vi "MarkerSkill.vi"(5 "SecondMostDangerous":bool, 7 "firstCall":bool, 8 "error in (no error)":errorcluster, 9 "Robot":refnum<class "Robot.lvclass">, 10 "Game":refnum<class "Game.lvclass">, 11 "MarkerSkill in":refnum<class "MarkerSkill.lvclass">) -> (0 "error out":errorcluster, 2 "Robot out":refnum<class "Robot.lvclass">, 3 "MarkerSkill out":refnum<class "MarkerSkill.lvclass">)   [LabVIEW 2020, in "MarkerSkill.lvclass"]
uses:
  MarkerSkill.lvclass
  Robot_class/Robot.lvclass
  Game_class/Game.lvclass
  Utilities_class/Utilities.lvclass
  Referee_class/command_interpreted.ctl
  Team_class/OffensivePlay.ctl
  Game_class/Game.lvclass/Game.ctl
  Team_class/Team.lvclass/Team.ctl
  Object_class/Object.lvclass/Object.ctl
  Parameters_class/Parameters.lvclass/Parameters.ctl
  Referee_class/Referee.lvclass/Referee.ctl
  Robot_class/Robot.lvclass/Robot.ctl
  Robot_class/roles.ctl
  Robot_class/Read role.vi
  Object_class/Read x.vi
  Object_class/Read y.vi
  Robot_class/Read id.vi
  <vilib>/Analysis/_algsub.llb/Real Vector Norm.vi
  Robot_class/Write dest_x.vi
  Robot_class/Write dest_y.vi
  Robot_class/Write dest_orientation.vi
  Robot_class/Write dest_vel.vi
  Robot_class/Read orientation.vi
  Game_class/Read BallRef.vi
  Game_class/Read Referee.vi
  Game_class/Read Parameters.lvclass.vi
  Parameters_class/Read DistanceStop.vi
  Referee_class/Read command_interpreted.vi
  Game_class/Read OffensiveTeam.vi
  Team_class/Read RobotRef.vi
  Game_class/Read EnemyRef.vi
  Game_class/Read Utilities.lvclass.vi
  Game_class/Read FieldRef.vi
  Parameters_class/Read Type of Marker.vi
  Team_class/Read OffensivePlay.vi
  Robot_class/Read dest_x.vi
  Robot_class/Read dest_y.vi
  Ball_class/Ball.lvclass
  Enemy_class/Enemy.lvclass
  Ally_class/Ally.lvclass
  Field_class/Field.lvclass
  Parameters_class/Parameters.lvclass
  Referee_class/Referee.lvclass
  <vilib>/Analysis/NI_AALPro.lvlib
panel:
  out "id do inimigo\nmais perigoso":u32
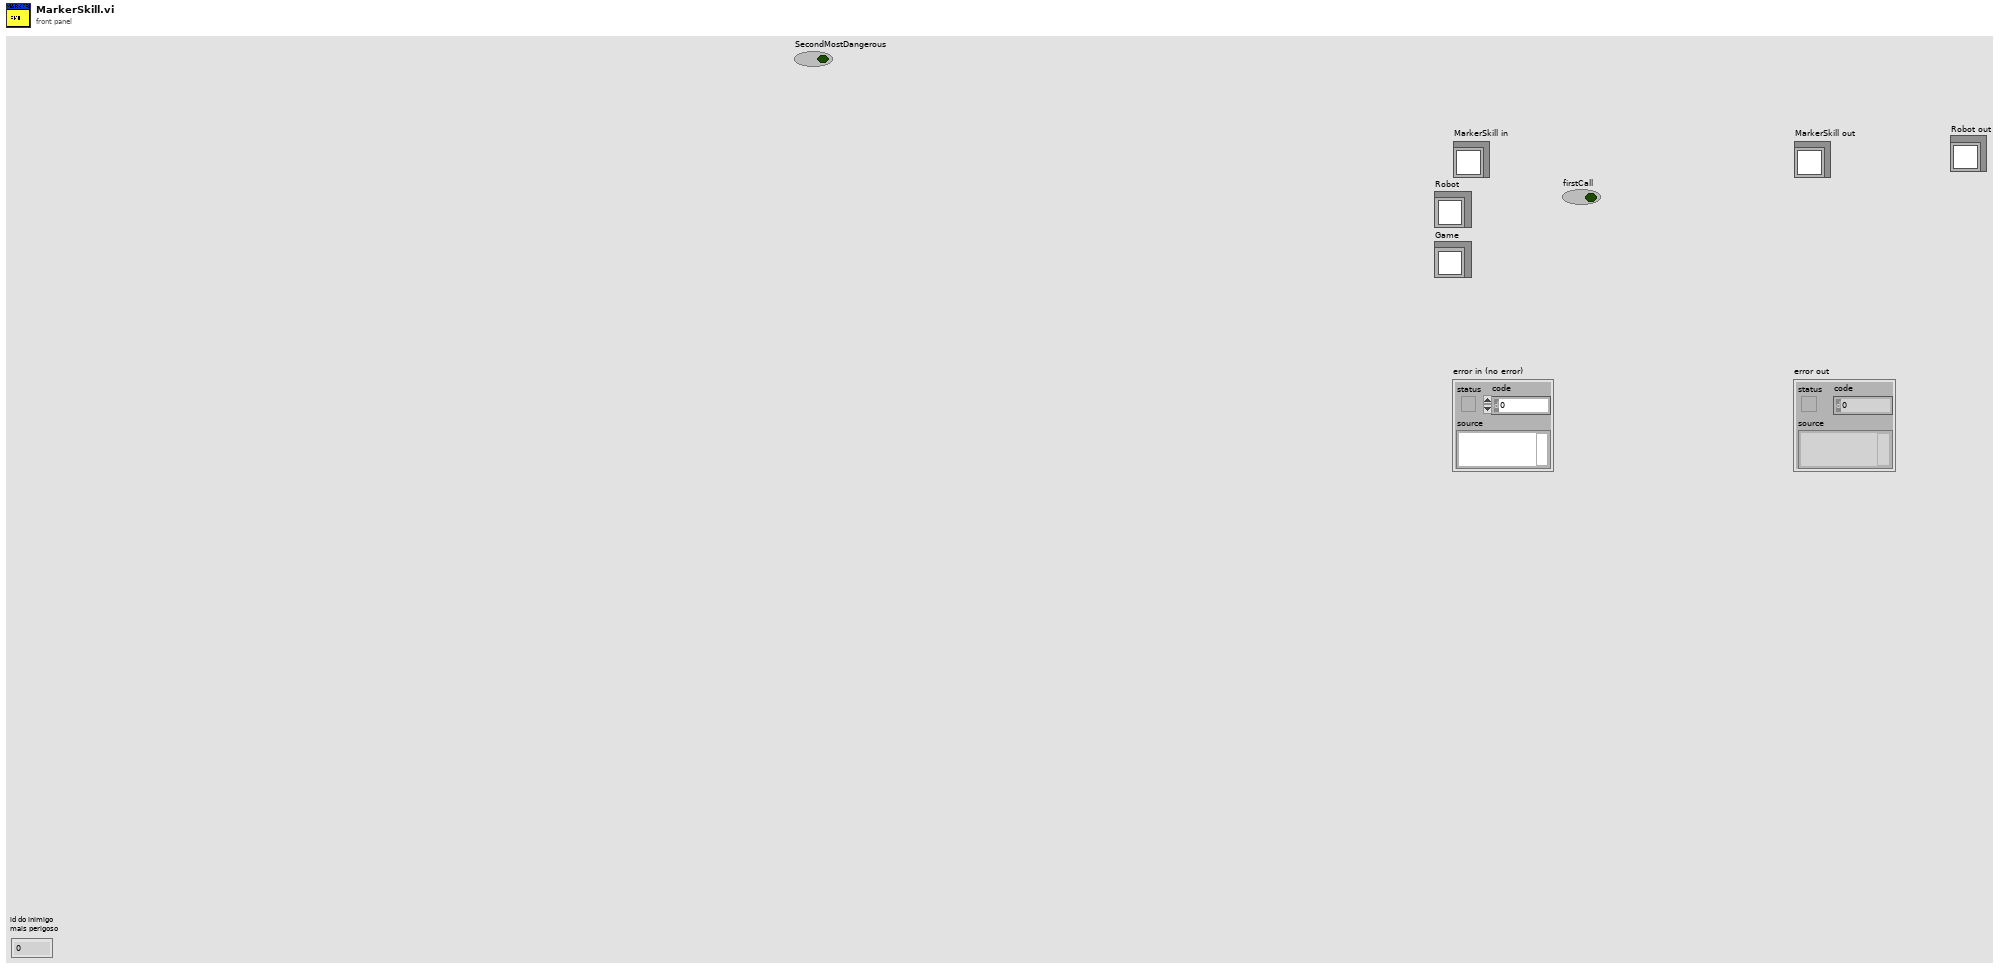
[diagram p1: front panel]
types:
  T1 = typedef "OffensivePlay.ctl" = enum16{"5RobotsPassGamePlay", "5PreparePassGame", "5RobotsKeeperGame", "KeeperPassToStriker", "5RobotsNormalGamePlay", "PrepareKeeperPass", "ACBPass", "ABCPass", "PrepareTriplePass", "TableWithStriker", "TableWith2ndStrikerPlay", "PrepareDoublePass", "PrepareRollToPass", "SimplePass", "PreparePass", "PassToStriker", "BallOutOfField", "PassTo2ndStriker", "StopOffensive", "Prepare Penalty Enemy", "EnemyPossessionAtEnemyField", "EnemyPossesionAtOurField", "TestPlay", "PreparePenaltyAlly", "KickPenaltyAlly", "PrepareKickoffAlly", "PrepareKickoffEnemy", "IndirectEnemy", "DirectEnemy", "PreparePassInGame1", "NormalGame", "DirectKick", "Pass", "Halt", "Timeout", "PassPlay", "PenaltyEnemy"}
  T2 = typedef "command_interpreted.ctl" = enum16{"Goal Ally", "Goal Enemy", "Ball Placement Enemy", "Ball Placement Ally", "Normal Half Time", "Extra Time  Break", "Extra Half Time", "None", "Post Game", "PKA Normal Start", "Prepare Kickoff Ally", "PKE Normal Start", "Prepare Kickoff Enemy", "Force Start", "Halt", "Timeout", "Prepare Penalty Ally", "Prepare Penalty Enemy", "PPA NormalStart", "PPE Normal Start", "Indirect Free Ally", "Direct Free Enemy", "Direct Free Ally", "Indirect Free Enemy", "Stop"}
  T3 = typedef "roles.ctl" = enum16{"SecondMarker", "5Robots5th", "PassBestReceiver", "5Robots4th", "5Robots3rd", "5Robots2nd", "5Robots1st", "PassBestRobot", "WaitPass", "ABCThirdKicker", "ABCFirstKicker", "ABCSecondKicker", "Tabler", "TableFinalizer", "PrepareRollToPassRoller", "PrepareRollToPassReceiver", "SimplePassRoll", "SimplePassRollReceiver", "PenaltyDefense", "PreparePassReceiver 2", "PreparePassReceiver 1", "PassObserver", "Timeout", "Goto", "ZigZag", "None", "BallOutOfField", "DefenderArea", "Duelist", "AttackerStop", "FollowAttacker", "KeeperRole", "KickPenalty", "AttackerAimGoal", "AttackerBlock", "Marker", "Halt", "Shoot", "PassKicker", "PassReceiver", "TestRole", "PenaltyAttacker"}
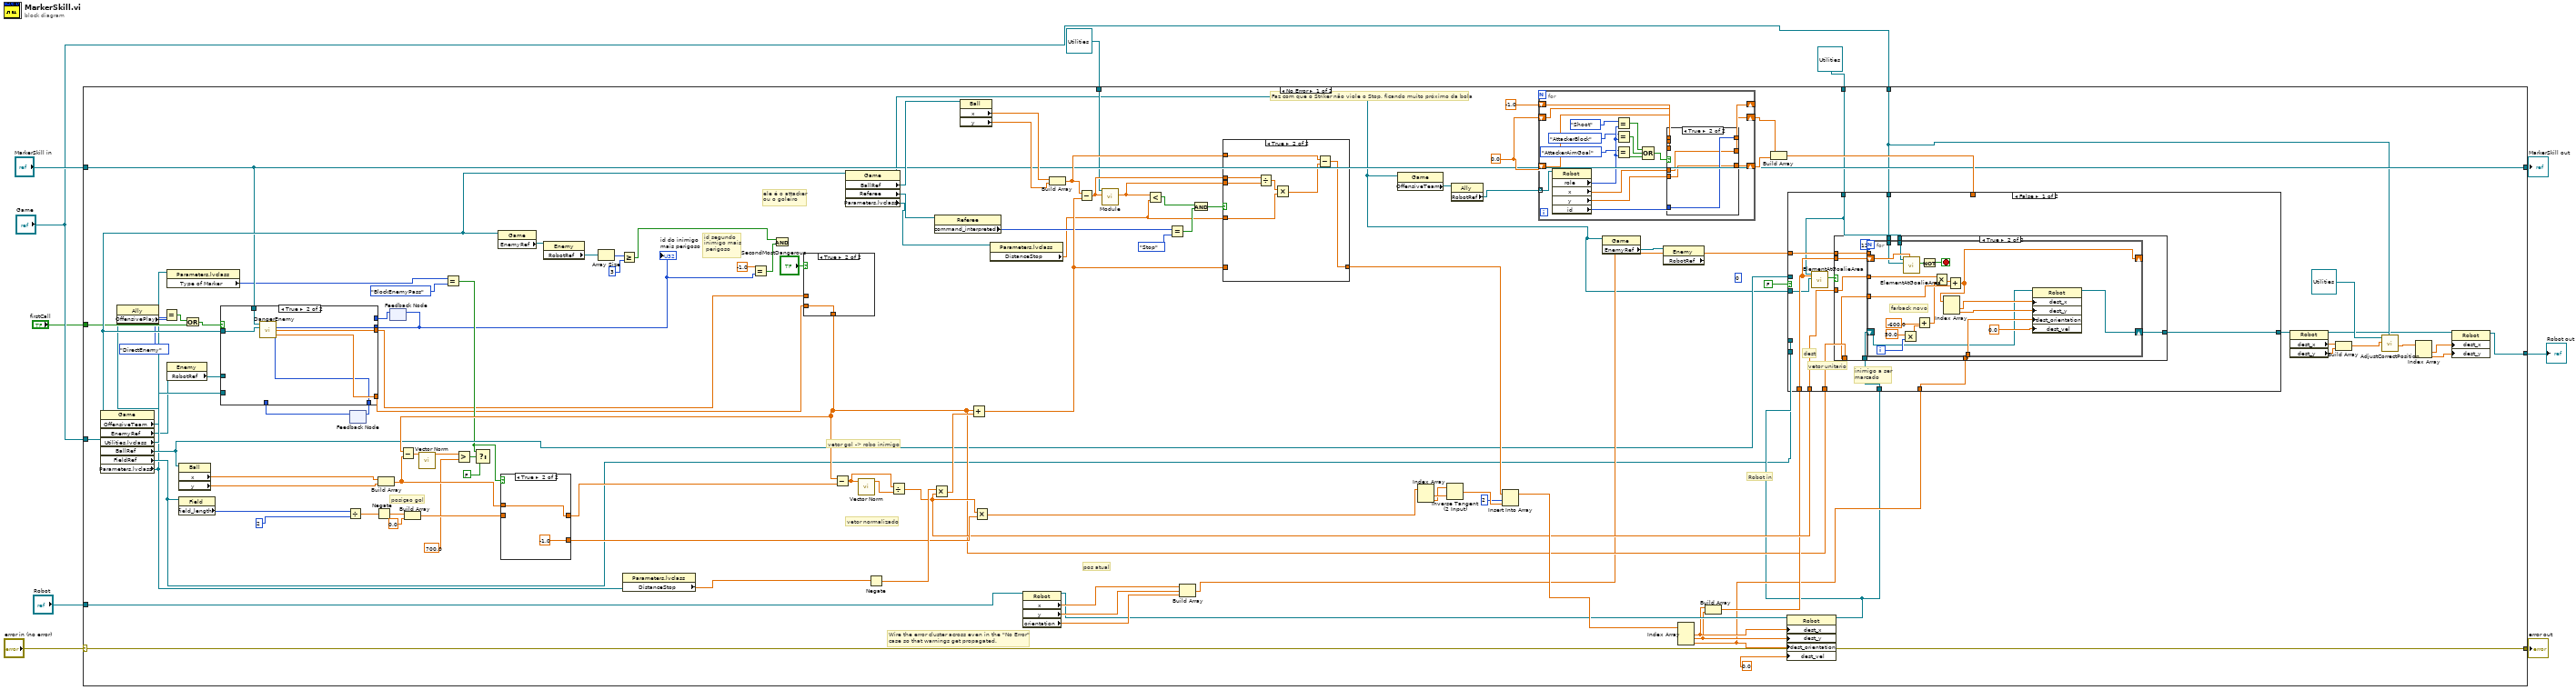
[diagram p0: block diagram]
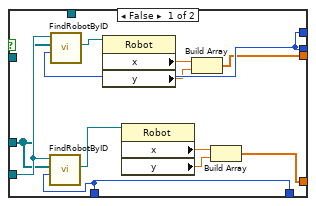
[diagram p2: hidden frame]
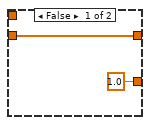
[diagram p7: hidden frame]
diagram:
  n1 = case shown="No Error" "error in (no error)" {
    selector: "error in (no error)" -> [w122 w222]
    tunnel: [w122 w222] -> w9
    tunnel: [w51 w221] -> w7
    tunnel: "MarkerSkill in" -> [w51 w221]
    tunnel: "Game" -> [w52 _]
    tunnel: "Robot" -> [w76 _]
    tunnel: refnum<class "Utilities.lvclass"> refnum ("Utilities in") -> [w48 _]
    tunnel: refnum<class "Utilities.lvclass"> refnum ("Utilities in") -> [w47 _]
    tunnel: "Game" -> [w26 _]
    tunnel: "firstCall" -> [w17 _]
    tunnel: [w22 _] -> w1
    frame No Error {
      (unwired) 0 ("y")
      w96 = 0.0
      # "id segundo \ninimigo mais\n perigoso"
      # "Robot in"
      # "ele é o attacker\nou o goleiro"
      # "Faz com que o Striker não viole o Stop, ficando muito próximo da bola"
      # "pos atual"
      # "vetor normalizado"
      # "vetor gol -> robo inimigo"
      # "posiçao gol"
      # "Wire the error cluster across even in the \"No Error\"\ncase so that warnings get propagated."
      n2 = property class="Game"(reference=w52) -> ("OffensiveTeam"=w16:refnum<class "Ally.lvclass">, "EnemyRef"=w32:refnum<class "Enemy.lvclass">, "Utilities.lvclass"=w33:refnum<class "Utilities.lvclass">, "BallRef"=w66:refnum<class "Ball.lvclass">, "FieldRef"=w54:refnum<class "Field.lvclass">, "Parameters.lvclass"=w12:refnum<class "Parameters.lvclass">)  [unwired: 1 in, 2 out]
      n3 = property class="Ally"(reference=w16) -> ("OffensivePlay"=w15:T1)  [unwired: 1 in, 2 out]
      n4 = Equal?(x=w15, y=OffensivePlay."DirectEnemy") -> (x = y?=w13:bool)
      n5 = property class="Enemy"(reference=w32) -> ("RobotRef"=w31:refnum<class "Robot.lvclass">[])  [unwired: 1 in, 2 out]
      n6 = property class="Parameters.lvclass"(reference=w12) -> ("Type of Marker"=w44:enum16{"BlockEnemyPass", "BlockOurGoal"})  [unwired: 1 in, 2 out]
      n7 = property class="Ball"(reference=w66) -> ("x"=w78:dbl, "y"=w77:dbl)  [unwired: 1 in, 2 out]
      n8 = property class="Field"(reference=w54) -> ("field_length"=w53:i32)  [unwired: 1 in, 2 out]
      n9 = Or(x=w13, y=w17) -> (x .or. y?=w18:bool)
      n10 = Divide(x=w53, y=u32 2) -> (x/y=w120:dbl)
      n11 = feedback #1() -> (w34:i32)  [unwired: 1 in]
      n12 = Negate(x=w120) -> (-x=w119:dbl)
      n13 = Build Array(w78, w77) -> (w89:dbl[])
      n14 = feedback #2() -> (w36:u32)  [unwired: 1 in]
      n15 = case shown="True" w18 {
        tunnel: [w133 w140] -> w37
        tunnel: [w127 w139] -> w38
        tunnel: [w123 w138] -> w39
        tunnel: w52 -> [_ w137]
        tunnel: w51 -> [_ w136]
        tunnel: w36 -> [w133 _]
        tunnel: [w131 w135] -> w35
        tunnel: w34 -> [w131 _]
        tunnel: w33 -> [w134 _]
        tunnel: w31 -> [w132 _]
        frame False {
          n16 = call "FindRobotByID.vi"("id"=w131, "RobotRef"=w132, "Utilities in"=w134) -> ("Robot"=w124:refnum<class "Robot.lvclass">)  [unwired: 5 in, 3 out]
          n17 = call "FindRobotByID.vi"("id"=w133, "RobotRef"=w132, "Utilities in"=w134) -> ("Robot"=w130:refnum<class "Robot.lvclass">)  [unwired: 5 in, 3 out]
          n18 = property class="Robot"(reference=w130) -> ("x"=w129:dbl, "y"=w128:dbl)  [unwired: 1 in, 2 out]
          n19 = property class="Robot"(reference=w124) -> ("x"=w126:dbl, "y"=w125:dbl)  [unwired: 1 in, 2 out]
          n20 = Build Array(w129, w128) -> (w127:dbl[])
          n21 = Build Array(w126, w125) -> (w123:dbl[])
        }
        frame True {
          n22 = call-dynamic "DangerEnemy.vi"("MarkerSkill in"=w136, "Game"=w137) -> ("id do inimigo\nmais perigoso"=w140:u32, "Pos do inimigo\nperigoso"=w139:dbl[], "id do segundo inimigo\nmais perigoso"=w135:i32, "Pos do segundo inimigo\nperigoso"=w138:dbl[])  [unwired: 6 in, 4 out]
        }
      }
      "id do inimigo\nmais perigoso" <- w37
      n23 = feedback-in #1(w35) -> ()
      n24 = feedback-in #2(w37) -> ()
      n25 = Build Array(w119, 0.0 ("element")) -> (w105:dbl[])
      n26 = Equal?(x=w44, y=enum16{"BlockEnemyPass", "BlockOurGoal"}."BlockEnemyPass" ("Type of Marker")) -> (x = y?=w45:bool)
      n27 = property class="Game"(reference=w52) -> ("EnemyRef"=w65:refnum<class "Enemy.lvclass">)  [unwired: 1 in, 2 out]
      n28 = case shown="True" w45 {
        tunnel: [w210 w211] -> w90
        tunnel: w105 -> [w210 _]
        tunnel: [1.0 -1.0] -> w101
        tunnel: w89 -> [_ w211]
        frame False {
        }
        frame True {
        }
      }
      n29 = property class="Enemy"(reference=w65) -> ("RobotRef"=w64:refnum<class "Robot.lvclass">[])  [unwired: 1 in, 2 out]
      n30 = Array Size(array=w64) -> (size(s)=w94:i32)
      n31 = Greater Or Equal?(x=w94, y=3) -> (x >= y?=w92:bool)
      n32 = property class="Parameters.lvclass"(reference=w12) -> ("DistanceStop"=w11:dbl)  [unwired: 1 in, 2 out]
      n33 = Equal?(x=-1.0, y=w37) -> (x = y?=w91:bool)
      n34 = And(x=w92, y=w91) -> ()  [unwired: 1 out]
      n35 = case shown="True" "SecondMostDangerous" {
        tunnel: w38 -> [w141 _]
        tunnel: w39 -> [_ w142]
        tunnel: [w141 w142] -> w80
        frame False {
        }
        frame True {
        }
      }
      n36 = Subtract(x=w80, y=w89) -> (x-y=w88:dbl[])
      n37 = call-poly <vilib>:"Vector Norm.vi"("Input Vector"=w88) -> ("norm"=w87:dbl)  [unwired: 9 in, 1 out]
      n38 = Greater?(x=w87, y=700.0) -> (0:w86:bool)
      n39 = Select(t=w45, s=w86, f=FALSE) -> ()  [unwired: 1 out]
      n40 = Subtract(x=w80, y=w90) -> (x-y=w116:dbl[])
      n41 = property class="Game"(reference=w52) -> (reference out=w40:refnum<class "Game.lvclass">, "BallRef"=w63:refnum<class "Ball.lvclass">, "Referee"=w60:refnum<class "Referee.lvclass">, "Parameters.lvclass"=w43:refnum<class "Parameters.lvclass">)  [unwired: 1 in, 1 out]
      n42 = call-poly <vilib>:"Vector Norm.vi"("Input Vector"=w116) -> ("norm"=w117:dbl)  [unwired: 9 in, 1 out]
      n43 = Negate(x=w11) -> (-x=w111:dbl)
      n44 = Divide(x=w116, y=w117) -> (x/y=w83:dbl[])
      n45 = Multiply(x=w111, y=w83) -> (x*y=w82:dbl[])
      n46 = property class="Referee"(reference=w60) -> ("command_interpreted"=w59:T2)  [unwired: 1 in, 2 out]
      n47 = property class="Ball"(reference=w63) -> ("x"=w62:dbl, "y"=w61:dbl)  [unwired: 1 in, 2 out]
      n48 = Add(x=w80, y=w82) -> (x+y=w107:dbl[])
      n49 = Multiply(x=w83, y=w101) -> (x*y=w102:dbl[])
      n50 = property class="Parameters.lvclass"(reference=w43) -> ("DistanceStop"=w42:dbl)  [unwired: 1 in, 2 out]
      n51 = property class="Robot"(reference=w76) -> (reference out=w72:refnum<class "Robot.lvclass">, "x"=w75:dbl, "y"=w74:dbl, "orientation"=w73:dbl)  [unwired: 1 in, 1 out]
      n52 = Build Array(w62, w61) -> (w106:dbl[])
      n53 = Subtract(x=w106, y=w107) -> (x-y=w50:dbl[])
      n54 = call "Module.vi"("2D vector"=w50, "Utilities in"=w47) -> ("Modulo"=w49:dbl)  [unwired: 7 in, 2 out]
      n55 = Less?(x=w49, y=w42) -> (x < y?=w110:bool)
      n56 = Equal?(x=w59, y=command_interpreted."Stop") -> (x = y?=w109:bool)
      n57 = Build Array(w75, w74, w73) -> (w79:dbl[])
      n58 = And(x=w110, y=w109) -> (x .and. y?=w108:bool)
      n59 = case shown="False" w108 {
        tunnel: [w213 w215] -> w104
        tunnel: w107 -> [w213 _]
        tunnel: w49 -> [_ w220]
        tunnel: w42 -> [_ w218]
        tunnel: w106 -> [_ w217]
        tunnel: w50 -> [_ w214]
        frame False {
        }
        frame True {
          n60 = Divide(x=w214, y=w220) -> (x/y=w219:dbl[])
          n61 = Multiply(x=w219, y=w218) -> (x*y=w216:dbl[])
          n62 = Subtract(x=w217, y=w216) -> (x-y=w215:dbl[])
        }
      }
      n63 = property class="Game"(reference=w40) -> ("OffensiveTeam"=w56:refnum<class "Ally.lvclass">)  [unwired: 1 in, 2 out]
      n64 = Index Array(array=w102) -> (element #1=w115:dbl, element #2=w114:dbl)  [unwired: 2 in]
      n65 = Inverse Tangent (2 Input)(1:w115, 2:w114) -> (0:w113:dbl)
      n66 = property class="Ally"(reference=w56) -> ("RobotRef"=w55:refnum<class "Robot.lvclass">[])  [unwired: 1 in, 2 out]
      n67 = Insert Into Array(array=w104, index=2, new element=w113) -> (w103:dbl[])
      n68 = for {
        tunnel: w55 -> [w153] mode=indexing
        shift-right: [w158] -> w99
        shift-left: w96 -> [w156]
        shift-right: [w157] -> w98
        shift-left: w96 -> [w155]
        shift-right: [w159] -> _
        shift-left: -1.0 -> [w154]
        n69 = property class="Robot"(reference=w153) -> ("role"=w149:T3, "x"=w152:dbl, "y"=w151:dbl, "id"=w150:i32)  [unwired: 1 in, 2 out]
        n70 = Equal?(x=roles."Shoot", y=w149) -> (x = y?=w145:bool)
        n71 = Equal?(x=roles."AttackerBlock", y=w149) -> (x = y?=w144:bool)
        n72 = Equal?(x=roles."AttackerAimGoal", y=w149) -> (x = y?=w143:bool)
        n73 = Compound Arithmetic op=OR(w145, w144, w143) -> (w160:bool)
        n74 = case shown="True" w160 {
          tunnel: w152 -> [_ w165]
          tunnel: w151 -> [_ w164]
          tunnel: w150 -> [_ w166]
          tunnel: [w161 w166] -> w159
          tunnel: [w163 w165] -> w158
          tunnel: [w162 w164] -> w157
          tunnel: w156 -> [w163 _]
          tunnel: w155 -> [w162 _]
          tunnel: w154 -> [w161 _]
          frame False {
          }
          frame True {
          }
        }
      }
      n75 = property class="Game"(reference=w40) -> ("EnemyRef"=w57:refnum<class "Enemy.lvclass">)  [unwired: 1 in, 2 out]
      n76 = property class="Enemy" props=["RobotRef"](reference=w57) -> ()  [unwired: 1 in, 3 out]
      n77 = Index Array(array=w103) -> (element #1=w71:dbl, element #2=w70:dbl, element #3=w69:dbl)  [unwired: 3 in]
      n78 = Build Array(w71, w70) -> (w81:dbl[])
      n79 = Build Array(w99, w98) -> (w97:dbl[])
      n80 = property class="Robot"(reference=w72, "dest_x"=w71, "dest_y"=w70, "dest_orientation"=w69, "dest_vel"=0.0) -> (reference out=w67:refnum<class "Robot.lvclass">)  [unwired: 1 in, 1 out]
      n81 = case shown="False" FALSE {
        tunnel: w67 -> [w174 _]
        tunnel: w67 -> [_ _]
        tunnel: w66 -> [_ _]
        tunnel: w97 -> [_ _]
        tunnel: w54 -> [_ _]
        tunnel: w83 -> [w176 _]
        tunnel: w80 -> [w177 _]
        tunnel: w81 -> [w172 _]
        tunnel: w69 -> [w175 _]
        tunnel: w79 -> [w173 _]
        tunnel: [w171 _] -> w29
        tunnel: w48 -> [w169 _]
        tunnel: w26 -> [w168 _]
        tunnel: w40 -> [w167 _]
        frame False {
          # "inimigo a ser\nmarcado"
          # "vetor unitario"
          # "dest"
          n82 = call-dynamic "ElementAtGoalieArea.vi"("Elemento pos."=w172, "Game"=w167, "Utilities in"=w169) -> ("Element at any goalkeeper area ?"=w170:bool)  [unwired: 5 in, 3 out]
          n83 = case shown="True" w170 {
            tunnel: w176 -> [_ w188]
            tunnel: w177 -> [_ w187]
            tunnel: w175 -> [_ w184]
            tunnel: [w178 w185] -> w171
            tunnel: w174 -> [w178 w186]
            tunnel: w173 -> [_ w183]
            tunnel: w172 -> [_ w182]
            tunnel: w169 -> [_ w180]
            tunnel: w168 -> [_ w179]
            frame False {
            }
            frame True {
              n84 = for {
                N: 12 -> [_]
                tunnel: w188 -> [w208]
                tunnel: w187 -> [w207]
                tunnel: w184 -> [w196]
                tunnel: w183 -> [_]
                shift-right: [w193] -> w185
                shift-left: w186 -> [w194]
                shift-right: [w199] -> _
                shift-left: w182 -> [w192]
                tunnel: w180 -> [w190]
                tunnel: w179 -> [w189]
                i -> [w202]
                stop <- w205 stop-if-true
                # "farback novo"
                n85 = Multiply(x=50.0, y=w202) -> (x*y=w201:dbl)
                n86 = call-dynamic "ElementAtGoalieArea.vi"("Elemento pos."=w192, "Game"=w189, "Utilities in"=w190) -> ("Element at any goalkeeper area ?"=w191:bool)  [unwired: 5 in, 3 out]
                n87 = Add(x=-600.0, y=w201) -> (x+y=w200:dbl)
                n88 = Not(x=w191) -> (.not. x?=w205:bool)
                n89 = Multiply(x=w208, y=w200) -> (x*y=w206:dbl[])
                n90 = Add(x=w206, y=w207) -> (x+y=w199:dbl[])
                n91 = Index Array(array=w199) -> (element #1=w198:dbl, element #2=w197:dbl)  [unwired: 2 in]
                n92 = property class="Robot"(reference=w194, "dest_x"=w198, "dest_y"=w197, "dest_orientation"=w196, "dest_vel"=0.0) -> (reference out=w193:refnum<class "Robot.lvclass">)  [unwired: 1 in, 1 out]
              }
            }
          }
        }
        frame True {
          # "FOLLOW ATTACKER"
        }
      }
      n93 = property class="Robot"(reference=w29) -> (reference out=w23:refnum<class "Robot.lvclass">, "dest_x"=w28:dbl, "dest_y"=w27:dbl)  [unwired: 1 in, 1 out]
      n94 = Build Array(w28, w27) -> (w25:dbl[])
      n95 = call "AdjustCorrectPosition.vi"("Game"=w26, "Position"=w25, "Utilities in"=refnum<class "Utilities.lvclass"> refnum) -> ("AdjustPosition"=w21:dbl[])  [unwired: 6 in, 2 out]
      n96 = Index Array(array=w21) -> (element #1=w20:dbl, element #2=w19:dbl)  [unwired: 2 in]
      n97 = property class="Robot"(reference=w23, "dest_x"=w20, "dest_y"=w19) -> (reference out=w22:refnum<class "Robot.lvclass">)  [unwired: 1 in, 1 out]
    }
    frame Error {
    }
  }
  "error out" <- w9
  "MarkerSkill out" <- w7
  "Robot out" <- w1
